vi "UI - Initiate Connection.vi"(8 "error in (no error)":errorcluster caption="错误输入（无错误）", 10 "Controller Address":string caption="控制器地址", 11 "Message Queue":refnum<queue> caption="消息队列") -> (0 "error out":errorcluster caption="错误输出", 1 "Connected?":bool caption="已连接？", 3 "dup Message Queue":refnum<queue> caption="消息队列副本")   [LabVIEW 2013]
uses:
  Message Queue/Message Cluster.ctl
  controls/Variable References.ctl
  Globals/Global - Configuration Options.vi
  Globals/Global - UI Stream and Variable Connections.vi
  Message Queue/Message Queue.lvlib
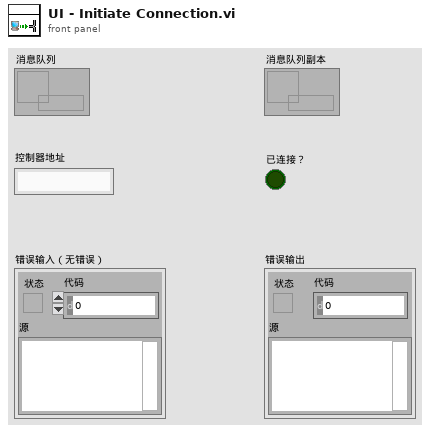
[diagram p1: front panel]
types:
  T1 = typedef "Message Queue.lvlib/Message Cluster.ctl" = cluster{"Message":string, "Message Data":variant}
  T2 = typedef "Variable References.ctl" = cluster{"CPU Usage":refnum<k21>, "Contiguous Memory":refnum<k21>, "Actual Loop Period":refnum<k21>, "Buffer Backlog":refnum<k21>, "Drive Space":refnum<k21>, "Number of Data Files":refnum<k21>, "System Time":refnum<k21>}
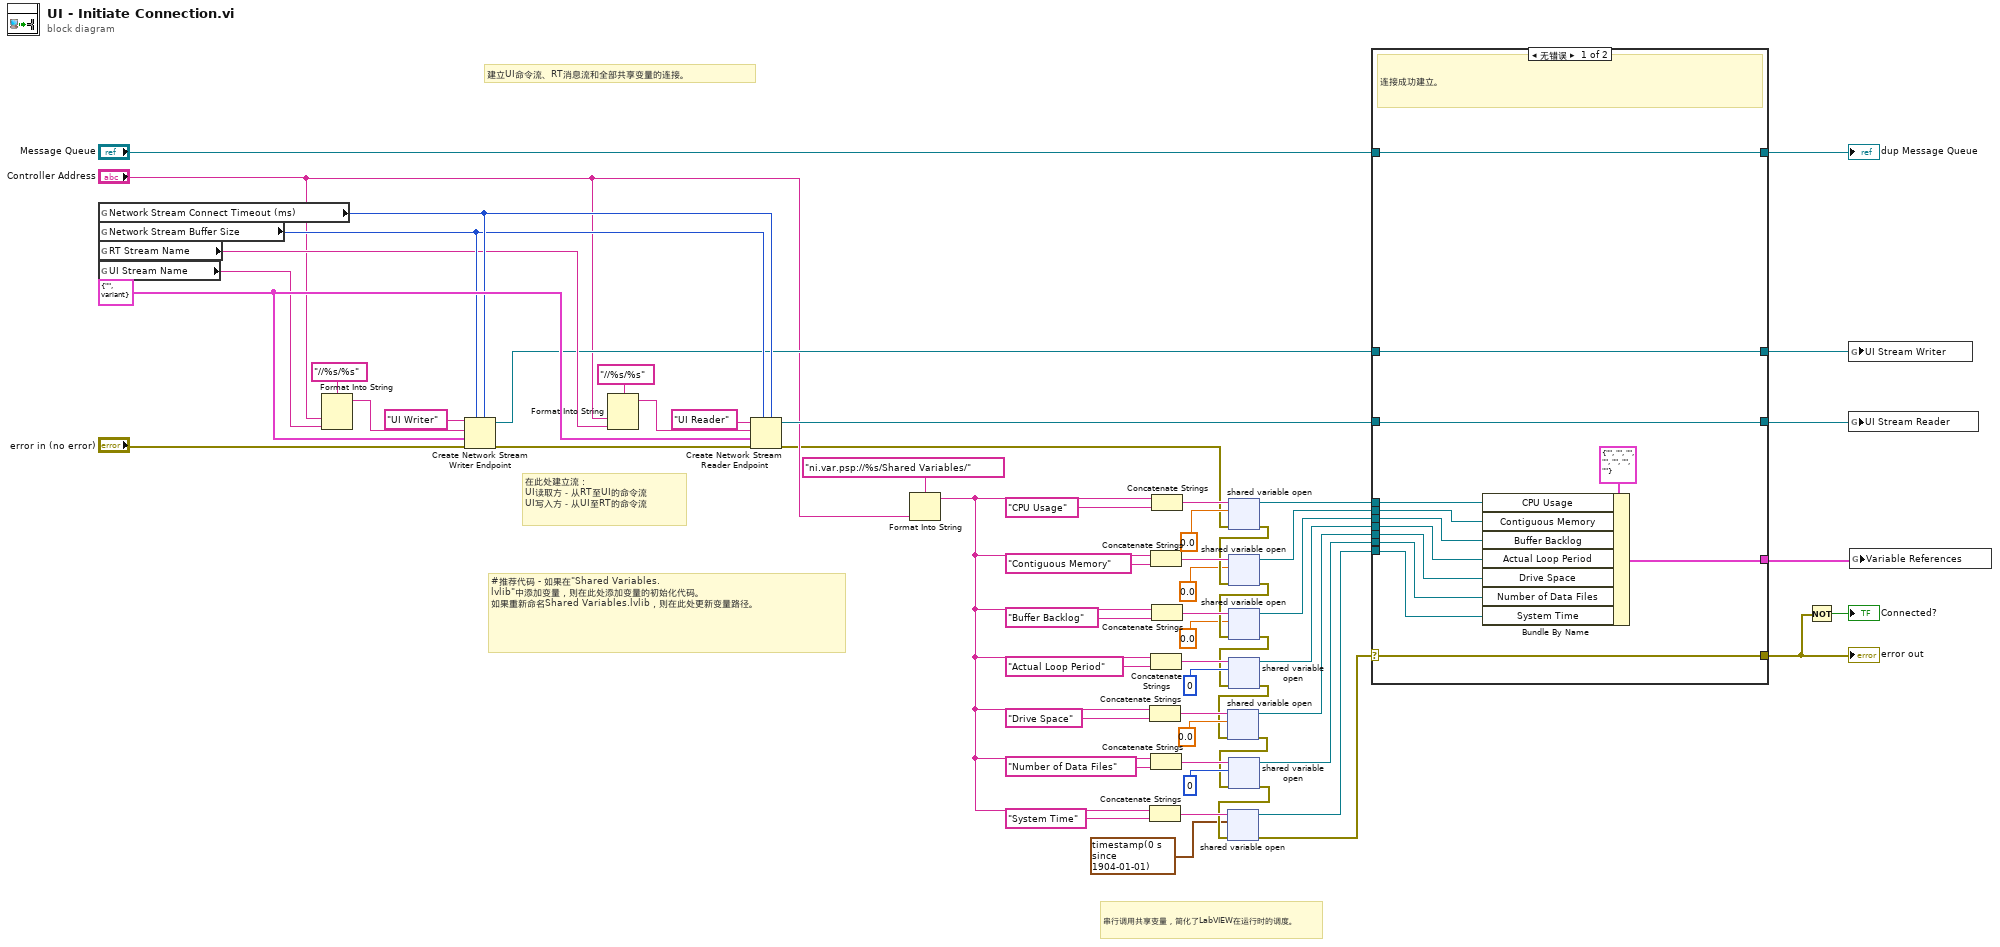
[diagram p0: block diagram]
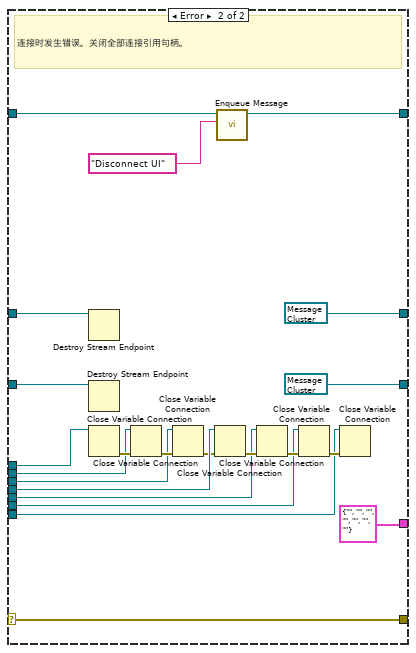
[diagram p2: hidden frame]
diagram:
  w55 = T1 {"Message"="", "Message Data"=variant} ("Message Cluster")
  # "建立UI命令流、RT消息流和全部共享变量的连接。"
  # "#推荐代码 - 如果在\"Shared Variables.lvlib\"中添加变量，则在此处添加变量的初始化代码。\n如果重新命名Shared Variables.lvlib，则在此处更新变量路径。"
  # "在此处建立流：\nUI读取方－从RT至UI的命令流\nUI写入方－从UI至RT的命令流"
  # "串行调用共享变量，简化了LabVIEW在运行时的调度。"
  n1 = global read "Global - Configuration Options.vi" "Network Stream Connect Timeout (ms)"() -> (w53:i32)
  n2 = global read "Global - Configuration Options.vi" "Network Stream Buffer Size"() -> (w13:i32)
  n3 = global read "Global - Configuration Options.vi" "RT Stream Name"() -> (w9:string)
  n4 = global read "Global - Configuration Options.vi" "UI Stream Name"() -> (w10:string)
  n5 = Format Into String(format string="//%s/%s", "Controller Address", w10) -> (resulting string=w7:string)  [unwired: 2 in, 1 out]
  n6 = Create Network Stream Writer Endpoint(5:w53, 7:w13, 8:"error in (no error)", 9:w55, 10:w7, 11:"UI Writer" ("reader name")) -> (0:w54:errorcluster, 3:w6:refnum<k21>)  [unwired: 1 in]
  n7 = Format Into String(format string="//%s/%s", "Controller Address", w9) -> (resulting string=w8:string)  [unwired: 2 in, 1 out]
  n8 = Create Network Stream Reader Endpoint(5:w53, 7:w13, 8:w54, 9:w55, 10:w8, 11:"UI Reader" ("writer name")) -> (0:w2:errorcluster, 3:w36:refnum<k21>)  [unwired: 1 in]
  n9 = Format Into String(format string="ni.var.psp://%s/Shared Variables/", "Controller Address") -> (resulting string=w5:string)  [unwired: 2 in, 1 out]
  n10 = Concatenate Strings(w5, "Drive Space") -> (w29:string)
  n11 = Concatenate Strings(w5, "System Time") -> (w20:string)
  n12 = Concatenate Strings(w5, "Contiguous Memory") -> (w48:string)
  n13 = Concatenate Strings(w5, "Actual Loop Period") -> (w44:string)
  n14 = Concatenate Strings(w5, "Number of Data Files") -> (w23:string)
  n15 = Concatenate Strings(w5, "CPU Usage") -> (w51:string)
  n16 = Concatenate Strings(w5, "Buffer Backlog") -> (w47:string)
  n17 = shared-variable-open(w51, w2, 0.0) -> (w40:refnum<k21>, w42:errorcluster)  [unwired: 1 in]
  n18 = shared-variable-open(w48, w42, 0.0) -> (w39:refnum<k21>, w41:errorcluster)  [unwired: 1 in]
  n19 = shared-variable-open(w47, w41, 0.0) -> (w38:refnum<k21>, w32:errorcluster)  [unwired: 1 in]
  n20 = shared-variable-open(w44, w32, u32 0) -> (w37:refnum<k21>, w28:errorcluster)  [unwired: 1 in]
  n21 = shared-variable-open(w29, w28, 0.0) -> (w27:refnum<k21>, w22:errorcluster)  [unwired: 1 in]
  n22 = shared-variable-open(w23, w22, u32 0) -> (w21:refnum<k21>, w19:errorcluster)  [unwired: 1 in]
  n23 = shared-variable-open(w20, w19, timestamp(0 s since 1904-01-01) ("time stamp")) -> (w17:refnum<k21>, w18:errorcluster)  [unwired: 1 in]
  n24 = case shown="无错误" w18 {
    selector: w18 -> [w62 w75]
    tunnel: w40 -> [w73 w92]
    tunnel: w39 -> [w72 w89]
    tunnel: w38 -> [w71 w90]
    tunnel: w37 -> [w70 w91]
    tunnel: w36 -> [w67 w95]
    tunnel: w6 -> [w68 w96]
    tunnel: [w69 T2 {"CPU Usage"="", "Contiguous Memory"="", "Actual Loop Period"="", "Buffer Backlog"="", "Drive Space"="", "Number of Data Files"="", "System Time"=""} ("Variable References")] -> w35
    tunnel: [w68 refnum<k21> refnum] -> w34
    tunnel: [w67 refnum<k21> refnum] -> w33
    tunnel: w27 -> [w66 w85]
    tunnel: w21 -> [w65 w83]
    tunnel: w17 -> [w64 w81]
    tunnel: "Message Queue" -> [w63 w78]
    tunnel: [w63 w76] -> w11
    tunnel: [w62 w75] -> w1
    frame No Error {
      # "连接成功建立。"
      n25 = Bundle By Name(cluster=T2 {"CPU Usage"="", "Contiguous Memory"="", "Actual Loop Period"="", "Buffer Backlog"="", "Drive Space"="", "Number of Data Files"="", "System Time"=""} ("Variable References"), "CPU Usage"=w73, "Contiguous Memory"=w72, "Buffer Backlog"=w71, "Actual Loop Period"=w70, "Drive Space"=w66, "Number of Data Files"=w65, "System Time"=w64) -> (w69:T2)
    }
    frame Error {
      # "连接时发生错误。关闭全部连接引用句柄。"
      n26 = Destroy Stream Endpoint(11:w96) -> ()  [unwired: 1 in, 1 out]
      n27 = Destroy Stream Endpoint(11:w95) -> ()  [unwired: 1 in, 1 out]
      n28 = Close Variable Connection(11:w92) -> (0:w93:errorcluster)  [unwired: 1 in]
      n29 = Close Variable Connection(8:w93, 11:w89) -> (0:w94:errorcluster)
      n30 = Close Variable Connection(8:w94, 11:w90) -> (0:w87:errorcluster)
      n31 = Close Variable Connection(8:w87, 11:w91) -> (0:w86:errorcluster)
      n32 = call "Enqueue Message.vi"("Message"="Disconnect UI", "Message Queue"=w78) -> ("dup Message Queue"=w76:refnum<queue>)  [unwired: 8 in, 1 out]
      n33 = Close Variable Connection(8:w86, 11:w85) -> (0:w84:errorcluster)
      n34 = Close Variable Connection(8:w84, 11:w83) -> (0:w82:errorcluster)
      n35 = Close Variable Connection(8:w82, 11:w81) -> ()  [unwired: 1 out]
    }
  }
  "error out" <- w1
  "dup Message Queue" <- w11
  n36 = Not(x=w1) -> (.not. x?=→"Connected?":bool)
  n37 = global write "Global - UI Stream and Variable Connections.vi" "UI Stream Writer"(w34) -> ()
  n38 = global write "Global - UI Stream and Variable Connections.vi" "UI Stream Reader"(w33) -> ()
  n39 = global write "Global - UI Stream and Variable Connections.vi" "Variable References"(w35) -> ()
